vi "build frame.vi"(8 "error in (no error)":errorcluster, 11 "frame data":T1) -> (0 "error out":errorcluster, 3 "<f> string":string)   [LabVIEW 2018, in "Data Parser.lvclass"]
uses:
  Data Parser.lvclass
  frame data.ctl
  frame title.ctl
  frame basic data.ctl
  frame o data.ctl
  frame bp data.ctl
  frame c data.ctl
  frame w data.ctl
  frame i data.ctl
  frame b data.ctl
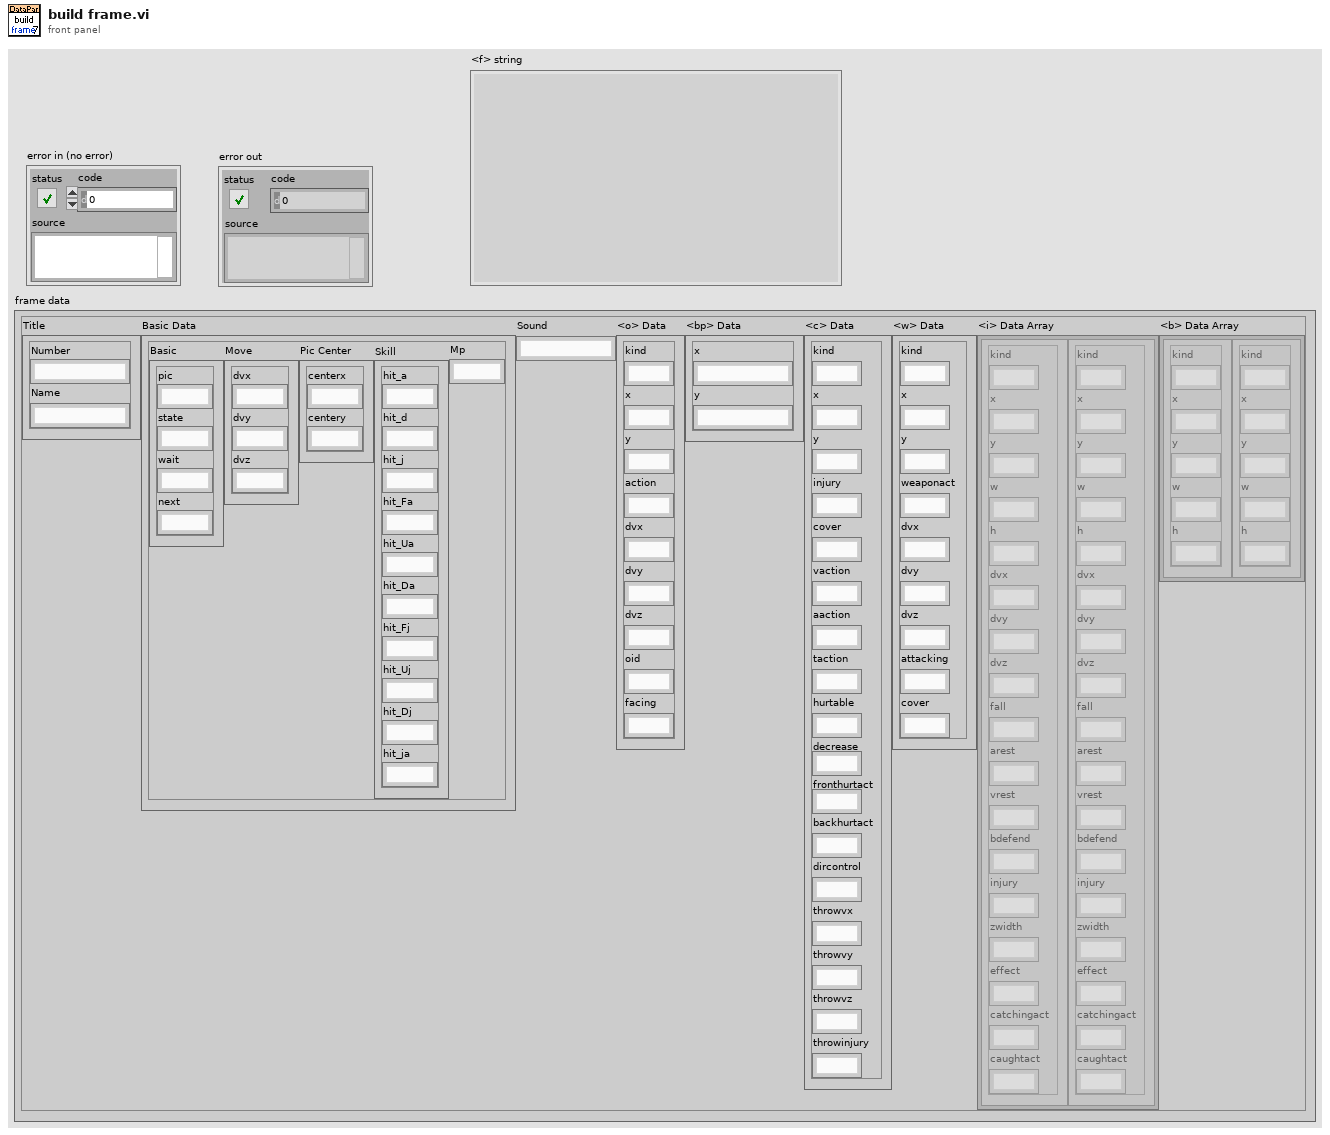
[diagram p1: front panel]
types:
  T1 = typedef "Data Parser.lvclass/frame data.ctl" = cluster{"Title":T2, "Basic Data":T3, "Sound":string, "<o> Data":T4, "<bp> Data":T5, "<c> Data":T6, "<w> Data":T7, "<i> Data Array":T8[], "<b> Data Array":T9[]}
  T2 = typedef "Data Parser.lvclass/frame title.ctl" = cluster{"Number":string, "Name":string}
  T3 = typedef "Data Parser.lvclass/frame basic data.ctl" = cluster{"Basic":cluster{"pic":string, "state":string, "wait":string, "next":string}, "Move":cluster{"dvx":string, "dvy":string, "dvz":string}, "Pic Center":cluster{"centerx":string, "centery":string}, "Skill":cluster{"hit_a":string, "hit_d":string, "hit_j":string, "hit_Fa":string, "hit_Ua":string, "hit_Da":string, "hit_Fj":string, "hit_Uj":string, "hit_Dj":string, "hit_ja":string}, "Mp":string}
  T4 = typedef "Data Parser.lvclass/frame o data.ctl" = cluster{"kind":string, "x":string, "y":string, "action":string, "dvx":string, "dvy":string, "dvz":string, "oid":string, "facing":string}
  T5 = typedef "Data Parser.lvclass/frame bp data.ctl" = cluster{"x":string, "y":string}
  T6 = typedef "Data Parser.lvclass/frame c data.ctl" = cluster{"kind":string, "x":string, "y":string, "injury":string, "cover":string, "vaction":string, "aaction":string, "taction":string, "hurtable":string, "decrease":string, "fronthurtact":string, "backhurtact":string, "dircontrol":string, "throwvx":string, "throwvy":string, "throwvz":string, "throwinjury":string}
  T7 = typedef "Data Parser.lvclass/frame w data.ctl" = cluster{"kind":string, "x":string, "y":string, "weaponact":string, "dvx":string, "dvy":string, "dvz":string, "attacking":string, "cover":string}
  T8 = typedef "Data Parser.lvclass/frame i data.ctl" = cluster{"kind":string, "x":string, "y":string, "w":string, "h":string, "dvx":string, "dvy":string, "dvz":string, "fall":string, "arest":string, "vrest":string, "bdefend":string, "injury":string, "zwidth":string, "effect":string, "catchingact":string, "caughtact":string}
  T9 = typedef "Data Parser.lvclass/frame b data.ctl" = cluster{"kind":string, "x":string, "y":string, "w":string, "h":string}
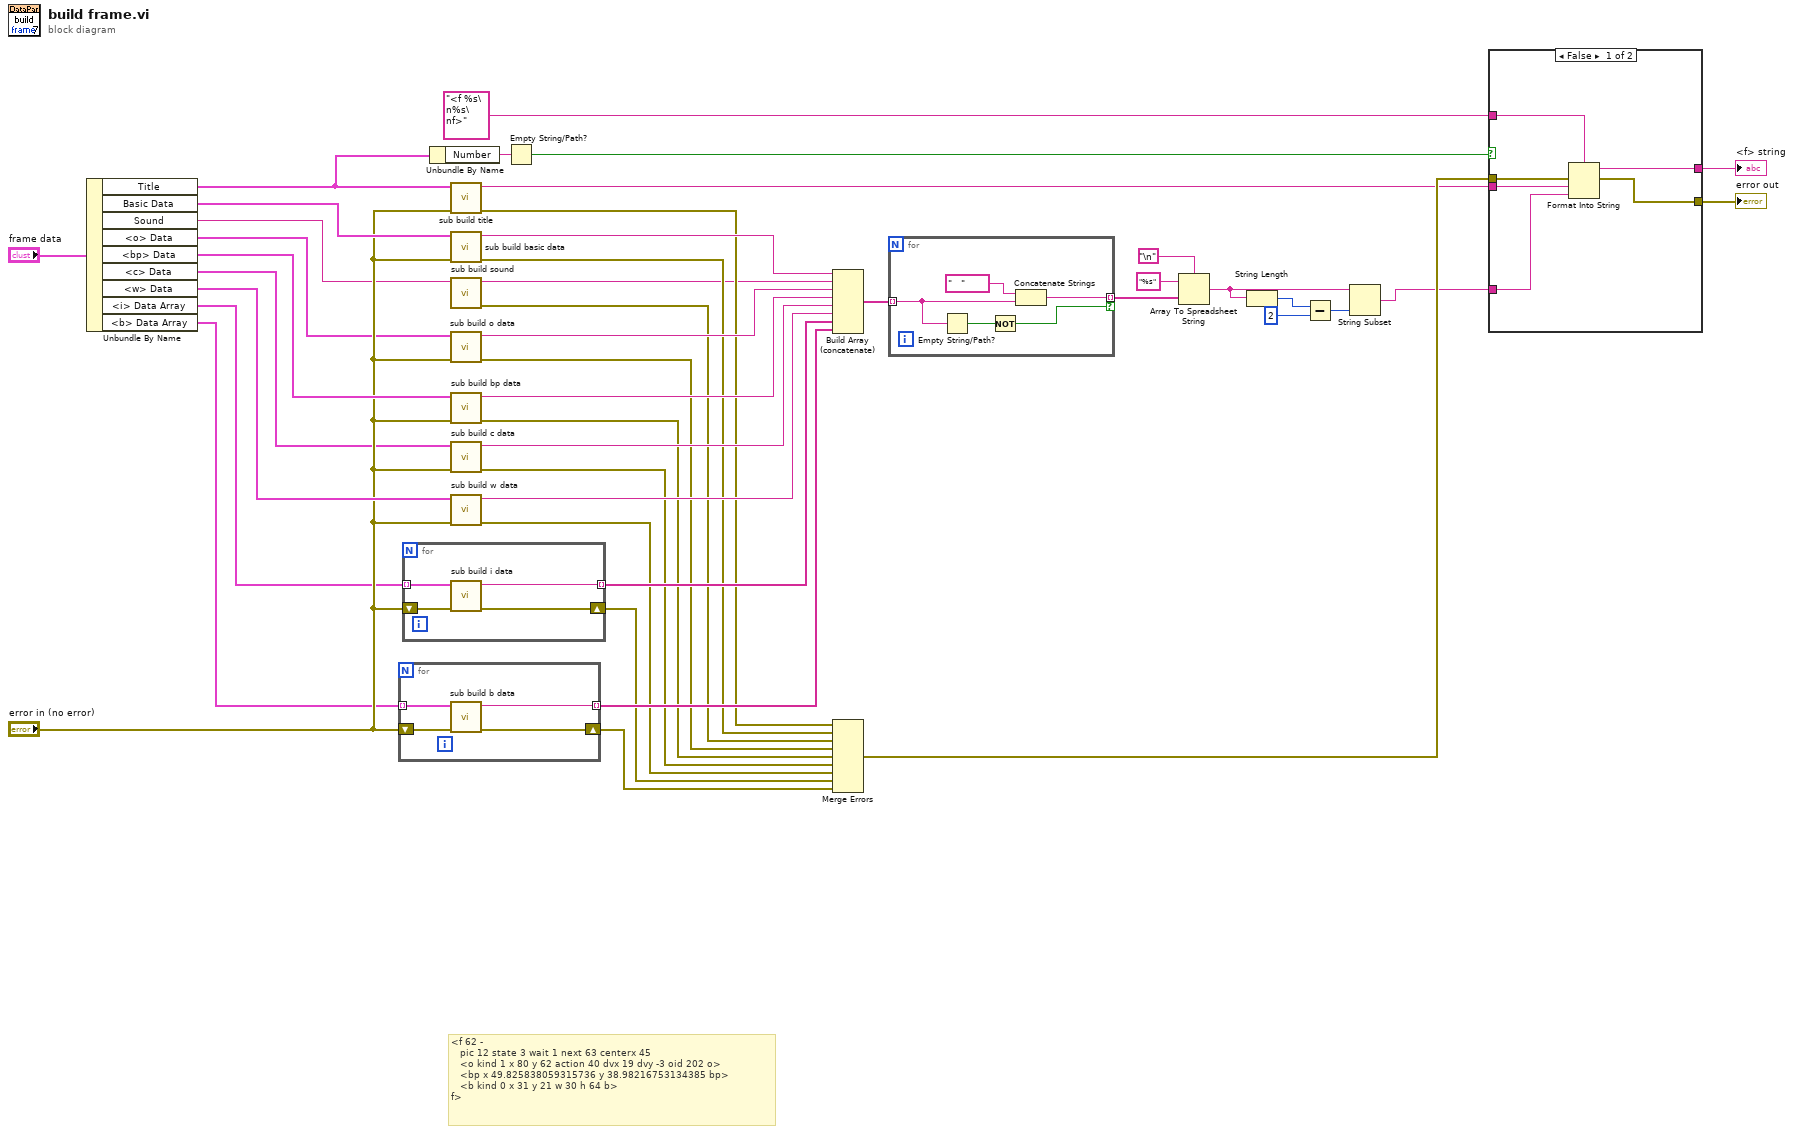
[diagram p0: block diagram]
diagram:
  # "<f 62 -\n   pic 12 state 3 wait 1 next 63 centerx 45\n   <o kind 1 x 80 y 62 action 40 dvx 19 dvy -3 oid 202 o>\n   <bp x 49.825838059315736 y 38.98216753134385 bp>\n   <b kind 0 x 31 y 21 w 30 h 64 b>\nf>"
  n1 = Unbundle By Name("frame data") -> ("Title"=w27:T2, "Basic Data"=w41:T3, "Sound"=w3:string, "<o> Data"=w6:T4, "<bp> Data"=w40:T5, "<c> Data"=w5:T6, "<w> Data"=w38:T7, "<i> Data Array"=w4:T8[], "<b> Data Array"=w17:T9[])
  n2 = for {
    tunnel: [w46] -> w18 mode=indexing
    shift-right: [w48] -> w7
    shift-left: "error in (no error)" -> [w47]
    tunnel: w17 -> [w45] mode=indexing
    n3 = call "sub build b data.vi"("error in"=w47, "<b> data"=w45) -> ("error out"=w48:errorcluster, "<b> string"=w46:string)  [unwired: 8 in]
  }
  n4 = for {
    tunnel: [w50] -> w19 mode=indexing
    shift-right: [w52] -> w8
    shift-left: "error in (no error)" -> [w51]
    tunnel: w4 -> [w49] mode=indexing
    n5 = call "sub build i data.vi"("error in"=w51, "<i> data"=w49) -> ("error out"=w52:errorcluster, "<i> string"=w50:string)  [unwired: 8 in]
  }
  n6 = Unbundle By Name(w27) -> ("Number"=w26:string)
  n7 = call "sub build title.vi"("error in"="error in (no error)", "frame title"=w27) -> ("error out"=w14:errorcluster, "title string"=w28:string)  [unwired: 8 in]
  n8 = call "sub build basic data.vi"("error in"="error in (no error)", "frame basic data"=w41) -> ("error out"=w13:errorcluster, "basic string"=w42:string)  [unwired: 8 in]
  n9 = call "sub build sound.vi"("sound"=w3) -> ("error out"=w1:errorcluster, "sound string"=w2:string)  [unwired: 9 in]
  n10 = call "sub build o data.vi"("error in"="error in (no error)", "<o> data"=w6) -> ("error out"=w12:errorcluster, "<o> string"=w16:string)  [unwired: 8 in]
  n11 = call "sub build bp data.vi"("error in"="error in (no error)", "<bp> data"=w40) -> ("error out"=w11:errorcluster, "<bp> string"=w39:string)  [unwired: 8 in]
  n12 = call "sub build c data.vi"("error in"="error in (no error)", "<c> data"=w5) -> ("error out"=w10:errorcluster, "<c> string"=w15:string)  [unwired: 8 in]
  n13 = call "sub build w data.vi"("error in"="error in (no error)", "<w> data"=w38) -> ("error out"=w9:errorcluster, "<w> string"=w37:string)  [unwired: 8 in]
  n14 = Empty String/Path?(string/path=w26) -> (empty?=w25:bool)
  n15 = Build Array (concatenate)(w42, w2, w16, w39, w15, w37, w19, w18) -> (w35:string[])
  n16 = Merge Errors(w14, w13, w1, w12, w11, w10, w9, w8, w7) -> (w30:errorcluster)
  n17 = for {
    tunnel: w35 -> [w55] mode=indexing
    tunnel: [w56] -> w34 mode=indexing if=w53
    n18 = Empty String/Path?(string/path=w55) -> (empty?=w54:bool)
    n19 = Not(x=w54) -> (.not. x?=w53:bool)
    n20 = Concatenate Strings("   " ("string"), w55) -> (w56:string)
  }
  n21 = Array To Spreadsheet String(delimiter (Tab)="\n", array=w34, 3:"%s" ("format string")) -> (spreadsheet string=w23:string)
  n22 = String Length(string=w23) -> (length=w22:i32)
  n23 = Subtract(x=w22, y=2) -> (x-y=w20:i32)
  n24 = String Subset(string=w23, length (rest)=w20) -> (substring=w24:string)  [unwired: 1 in]
  n25 = case shown="False" w25 {
    tunnel: "<f %s\n%s\nf>" ("format string") -> [w63 _]
    tunnel: w24 -> [w62 _]
    tunnel: [w61 _] -> w32
    tunnel: w30 -> [w60 w64]
    tunnel: [w59 w64] -> w29
    tunnel: w28 -> [w58 _]
    frame False {
      n26 = Format Into String(format string=w63, error in=w60, w58, w62) -> (resulting string=w61:string, error out=w59:errorcluster)  [unwired: 1 in]
    }
    frame True {
    }
  }
  "<f> string" <- w32
  "error out" <- w29
